vi "Initialize Hardware.vi"(7 "RT config file":path, 8 "error in":errorcluster, 11 "device parameters":T5) -> (0 "error out":errorcluster, 3 "RT handles":T4, 5 "device information":T1)   [LabVIEW 2020, in "Communication Bus Template Engine.lvlib" / "Custom Device.lvlib"]
uses:
  Custom Device.lvlib
  Shared/Device Parameters.ctl
  Shared/Initialization Method.ctl
  Hardware Handles.ctl
  Device Information.ctl
  Hardware Direction and Channels.ctl
  Shared/Direction Capability.ctl
  <instrlib>/BTICardLib/Private/Initialize By Card Number and Core Number.vi
  <instrlib>/BTICardLib/Private/Initialize By Slot Number and Core Number.vi
  <instrlib>/BTICardLib/Private/IO/Action-Status/Write External LED.vi
  <instrlib>/BTICardLib/Private/Configure All From XML.vi
  <instrlib>/BTI429Lib/Private/Core/Action-Status/Start All Channels.vi
  <instrlib>/BTICardLib/BTICardLV.lvlib
  <instrlib>/BTI429Lib/BTI429LV.lvlib
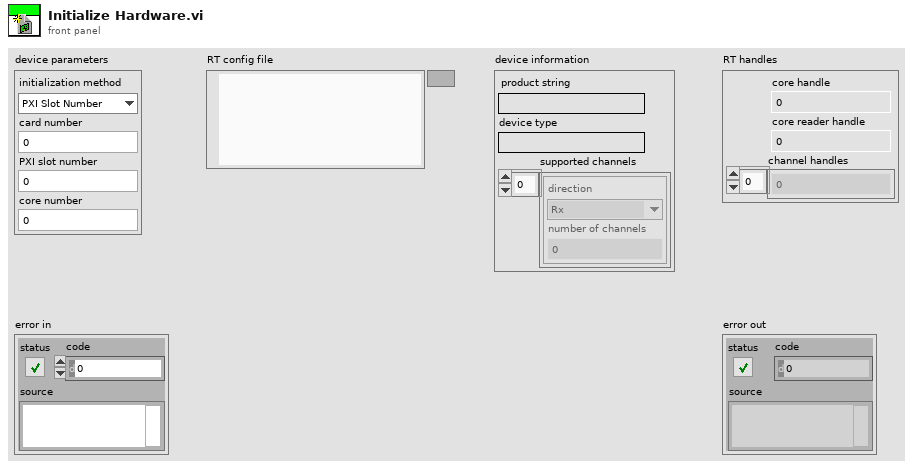
[diagram p1: front panel]
types:
  T1 = typedef "Communication Bus Template Engine.lvlib/Custom Device.lvlib/Device Information.ctl" = cluster{"product string":string, "device type":string, "supported channels":T2[]}
  T2 = typedef "Communication Bus Template Engine.lvlib/Custom Device.lvlib/Hardware Direction and Channels.ctl" = cluster{"direction":T3, "number of channels":u16}
  T3 = typedef "Direction Capability.ctl" = enum16{"Rx", "Tx", "Rx/Tx"}
  T4 = typedef "Communication Bus Template Engine.lvlib/Custom Device.lvlib/Hardware Handles.ctl" = cluster{"core handle":u64, "core reader handle":u64, "channel handles":u64[]}
  T5 = typedef "Device Parameters.ctl" = cluster{"initialization method":T6, "card number":i32, "PXI slot number":i32, "core number":i32}
  T6 = typedef "Initialization Method.ctl" = enum16{"PXI Slot Number", "Card Number"}
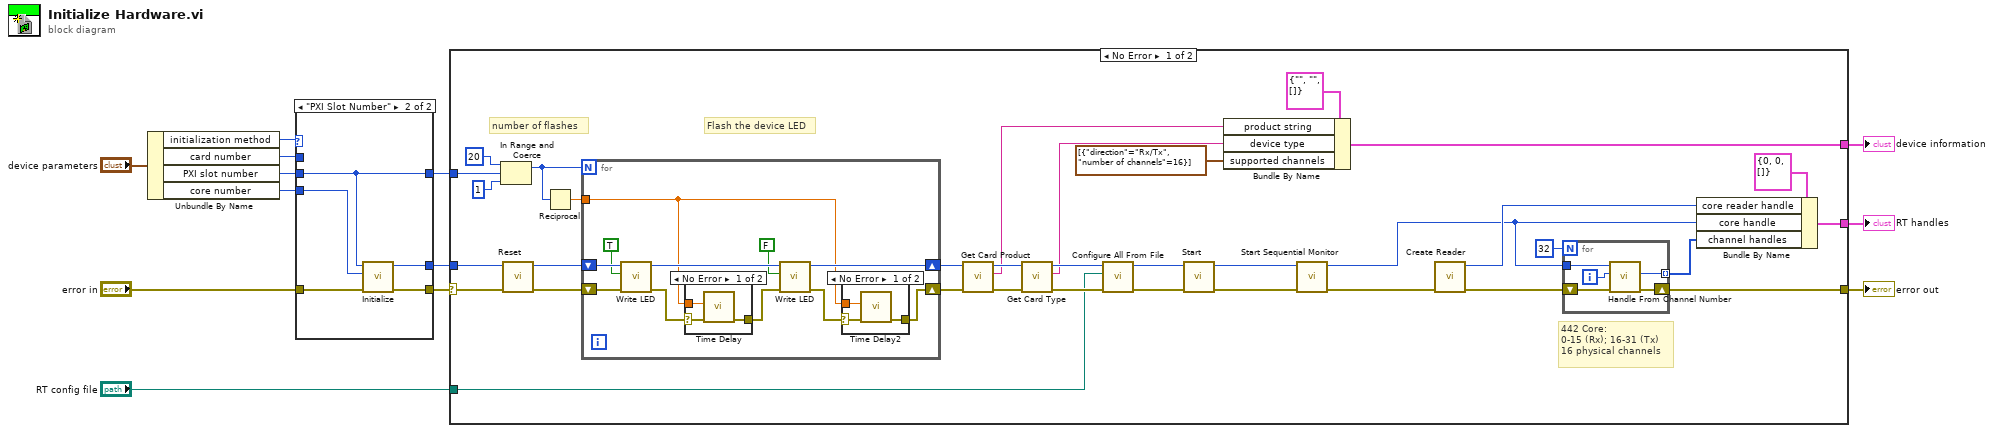
[diagram p0: block diagram]
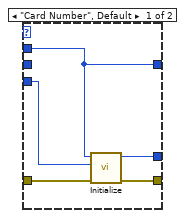
[diagram p5: hidden frame]
diagram:
  n1 = Unbundle By Name("device parameters") -> ("initialization method"=w13:T6, "card number"=w12:i32, "PXI slot number"=w11:i32, "core number"=w8:i32)
  n2 = case shown="\"PXI Slot Number\"" w13 {
    tunnel: [w18 w23] -> w6
    tunnel: [w17 w22] -> w9
    tunnel: w12 -> [w14 _]
    tunnel: "error in" -> [w16 w21]
    tunnel: w11 -> [_ w19]
    tunnel: w8 -> [w15 w20]
    tunnel: [w14 w19] -> w5
    frame "Card Number", Default {
      n3 = call-poly <instrlib>:"Initialize.vi"("error in (no error)"=w16, "core number"=w15, "card number"=w14) -> ("error out"=w17:errorcluster, "core handle out"=w18:u64)  [unwired: 7 in]
    }
    frame "PXI Slot Number" {
      n4 = call-poly <instrlib>:"Initialize.vi"("error in (no error)"=w21, "core number"=w20, "slot number"=w19) -> ("error out"=w22:errorcluster, "core handle out"=w23:u64)  [unwired: 7 in]
    }
  }
  n5 = case shown="No Error" w9 {
    selector: w9 -> [w57 w82]
    tunnel: w6 -> [w56 _]
    tunnel: w5 -> [w53 _]
    tunnel: [w31 _] -> w4
    tunnel: [w29 _] -> w3
    tunnel: [w28 w82] -> w2
    tunnel: "RT config file" -> [w25 _]
    frame No Error {
      # "442 Core:\n0-15 (Rx); 16-31 (Tx)\n16 physical channels"
      # "number of flashes"
      # "Flash the device LED"
      n6 = In Range and Coerce(upper limit=20 ("x"), x=w53, lower limit=1) -> (coerced(x)=w49:i32)  [unwired: 1 out]
      n7 = call <instrlib>:"Reset.vi"("error in (no error)"=w57, "core handle in"=w56) -> ("error out"=w55:errorcluster, "core handle out"=w54:u64)  [unwired: 8 in]
      n8 = Reciprocal(x=w49) -> (1/x=w50:dbl)
      n9 = for {
        N: w49 -> [_]
        shift-right: [w72] -> w46
        shift-left: w54 -> [w71]
        shift-right: [w66] -> w45
        shift-left: w55 -> [w70]
        tunnel: w50 -> [w63]
        n10 = call-poly <instrlib>:"Write LED.vi"("error in (no error)"=w70, "LED state"=TRUE, "core handle in"=w71) -> ("error out"=w65:errorcluster, "core handle out"=w73:u64)  [unwired: 7 in]
        n11 = case shown="No Error" w65 {
          selector: w65 -> [w76 w77]
          tunnel: [w75 w77] -> w64
          tunnel: w63 -> [w74 _]
          frame No Error {
            n12 = call "Time Delay"("error in (no error)"=w76, "Delay Time (s)"=w74) -> ("error out"=w75:errorcluster)  [unwired: 9 in]
          }
          frame Error {
          }
        }
        n13 = call-poly <instrlib>:"Write LED.vi"("error in (no error)"=w64, "LED state"=FALSE, "core handle in"=w73) -> ("error out"=w67:errorcluster, "core handle out"=w72:u64)  [unwired: 7 in]
        n14 = case shown="No Error" w67 {
          selector: w67 -> [w80 w81]
          tunnel: [w79 w81] -> w66
          tunnel: w63 -> [w78 _]
          frame No Error {
            n15 = call "Time Delay2"("error in (no error)"=w80, "Delay Time (s)"=w78) -> ("error out"=w79:errorcluster)  [unwired: 9 in]
          }
          frame Error {
          }
        }
      }
      n16 = call <instrlib>:"Get Card Product.vi"("error in (no error)"=w45, "core handle in"=w46) -> ("error out"=w47:errorcluster, "product string out"=w35:string, "core handle out"=w48:u64)  [unwired: 7 in]
      n17 = call <instrlib>:"Get Card Type.vi"("error in (no error)"=w47, "core handle in"=w48) -> ("error out"=w36:errorcluster, "type string out"=w34:string, "core handle out"=w37:u64)  [unwired: 7 in]
      n18 = call-poly <instrlib>:"Configure All From File.vi"("error in (no error)"=w36, "configuration file path"=w25, "core handle in"=w37) -> ("error out"=w39:errorcluster, "core handle out"=w40:u64)  [unwired: 7 in]
      n19 = call-poly <instrlib>:"Start.vi"("error in (no error)"=w39, "core handle in"=w40) -> ("error out"=w43:errorcluster, "core handle out"=w42:u64)  [unwired: 8 in]
      n20 = Bundle By Name(cluster=T1 {"product string"="", "device type"="", "supported channels"=[]} ("hardware information"), "product string"=w35, "device type"=w34, "supported channels"=T2[] [{"direction"=enum."Rx/Tx", "number of channels"=16}]) -> (w31:T1)
      n21 = call <instrlib>:"Start Sequential Monitor.vi"("error in (no error)"=w43, "core handle in"=w42) -> ("error out"=w44:errorcluster, "core handle out"=w24:u64)  [unwired: 8 in]
      n22 = call <instrlib>:"Create Reader.vi"("error in (no error)"=w44) -> ("error out"=w38:errorcluster, "core reader handle out"=w26:u64)  [unwired: 9 in]
      n23 = for {
        N: 32 -> [_]
        shift-right: [w59] -> w28
        shift-left: w38 -> [w62]
        tunnel: [w60] -> w27 mode=indexing
        tunnel: w24 -> [w58]
        i -> [w61]
        n24 = call <instrlib>:"Handle From Channel Number.vi"("error in (no error)"=w62, "channel number"=w61, "core handle in"=w58) -> ("error out"=w59:errorcluster, "channel handle out"=w60:u64)  [unwired: 6 in, 1 out]
      }
      n25 = Bundle By Name(cluster=T4 {"core handle"=0, "core reader handle"=0, "channel handles"=[]} ("hardware handles"), "core reader handle"=w26, "core handle"=w24, "channel handles"=w27) -> (w29:T4)
    }
    frame Error {
    }
  }
  "RT handles" <- w3
  "error out" <- w2
  "device information" <- w4
